vi "bigcryo_Harry-IcT - v2.vi"(10 "Stop":bool, 11 "Measure":bool) -> ()   [LabVIEW 2019]
uses:
  Components/Global 2.vi
  <vilib>/Utility/file.llb/Read From Spreadsheet File (DBL).vi
panel:
  out "SampleTemp":dbl
  in  "Settle Time (s)":dbl=60.0
  in  "Step/Ramp":bool=TRUE
  in  "T Rate (K/min)":dbl=0.1
  out "dV/dI-I":cluster{dbl[], dbl[]}(graph) caption="XY Graph"
  out "I-V":cluster{dbl[], dbl[]}(graph) caption="XY Graph"
  out "Status":string="Measuring..."
  in  "Keithley":refnum<visa-resource-name>="GPIB1::20::INSTR"
  in  "Delay [sec]":dbl=0.002 format="%#_6e"
  in  "Compliance [V] 2":dbl=10.0 format="%#_6f"
  in  "Delta [A]":dbl=1e-05 format="%#_6e"
  in  "Abort Conductance":bool
  in  "Step [A]":dbl=1e-05 format="%#_6e"
  in  "I-Max [A]":dbl=0.002 format="%#_6e"
  in  "Arm Conductance":bool
  in  "Directory Output":string="C:\\User Data\\hlb54\\210111_42B\\JJ1\\IcT_test"
  in  "Minicryo":bool=TRUE
  in  "Field and rate":dbl[][](array[numeric])
  out "?":refnum<visa-resource-name>="GPIB1::20::INSTR"
  out "Iteration?":i32=401
  in  "Start Temp (K)":dbl=2.0 format="%#_7f"
  in  "T Step (K)":dbl=0.01
  out "T Aim":dbl=2.02
  in  "Stop Temp (K)":dbl=2.1
  # "Step"
  # "Ramp"
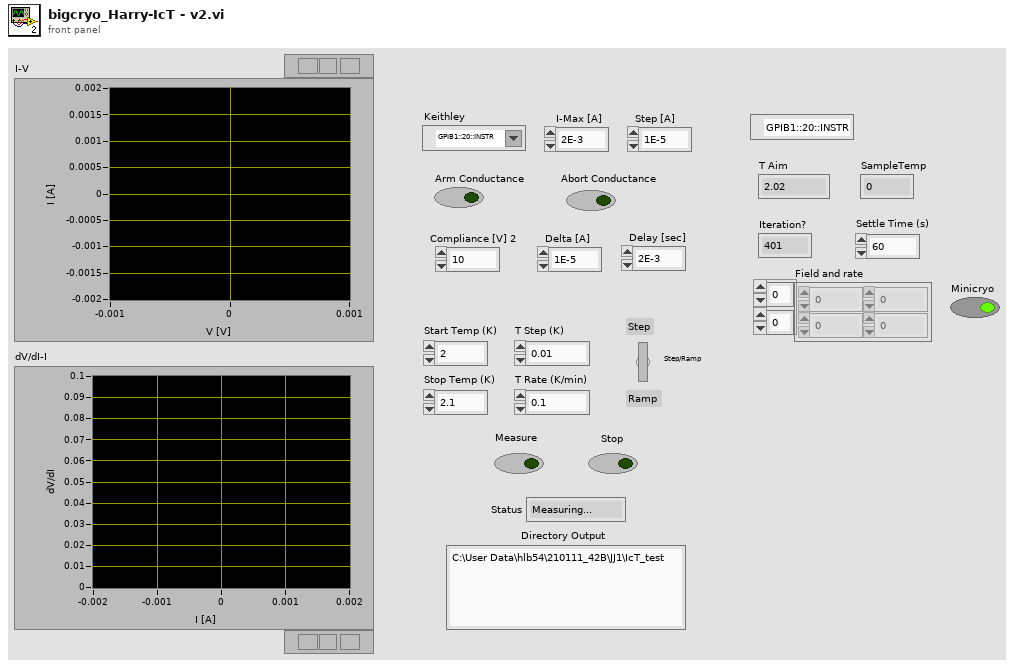
[diagram p1: front panel]
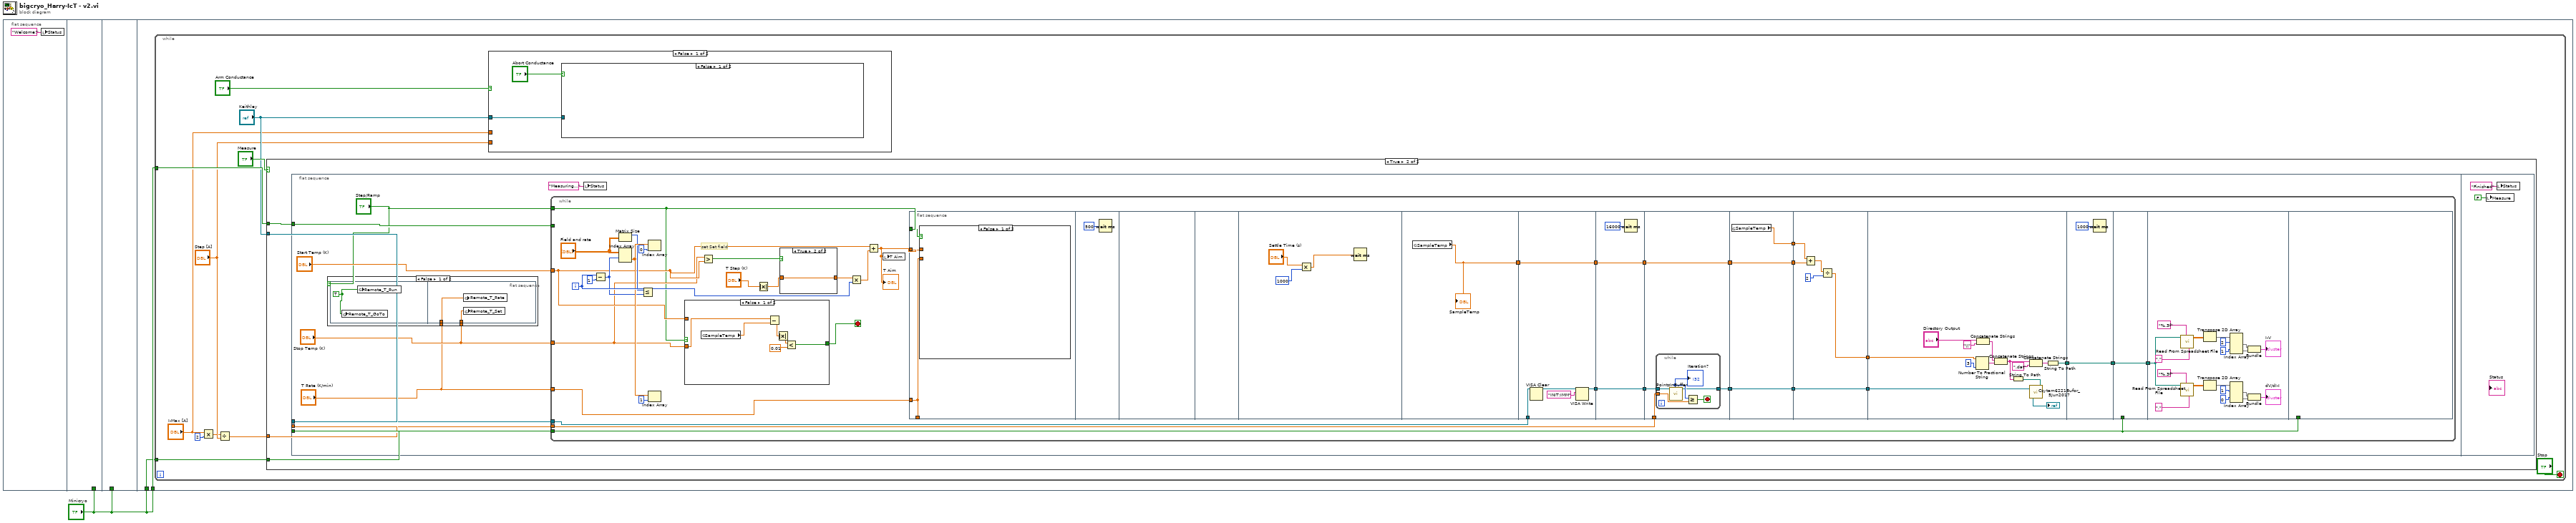
[diagram p0: block diagram]
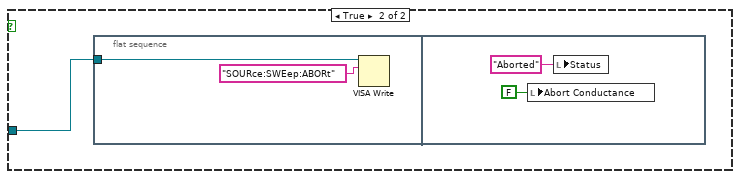
[diagram p2: hidden frame]
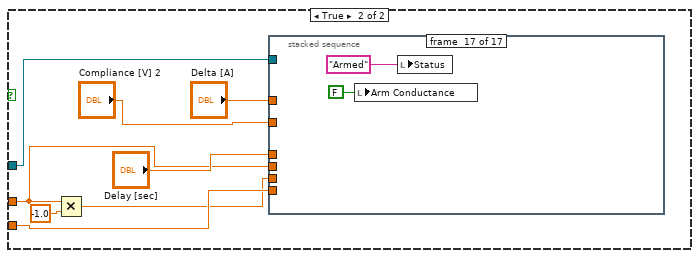
[diagram p3: hidden frame]
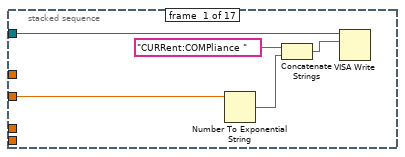
[diagram p4: hidden frame]
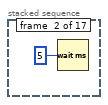
[diagram p5: hidden frame]
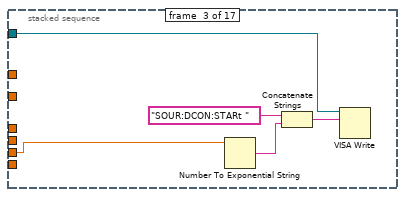
[diagram p6: hidden frame]
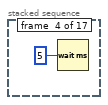
[diagram p7: hidden frame]
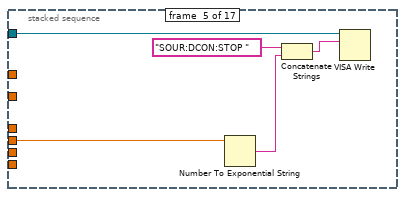
[diagram p8: hidden frame]
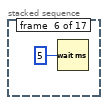
[diagram p9: hidden frame]
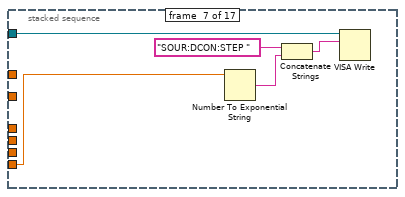
[diagram p10: hidden frame]
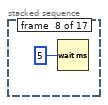
[diagram p11: hidden frame]
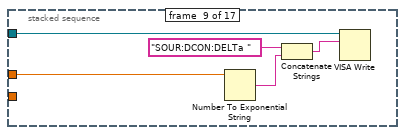
[diagram p12: hidden frame]
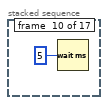
[diagram p13: hidden frame]
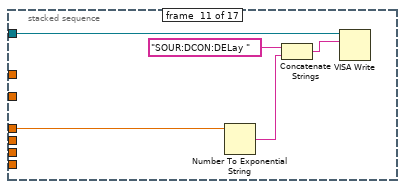
[diagram p14: hidden frame]
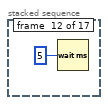
[diagram p15: hidden frame]
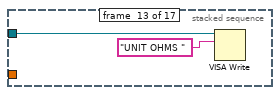
[diagram p16: hidden frame]
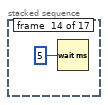
[diagram p17: hidden frame]
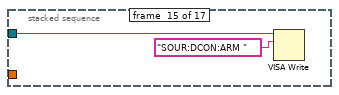
[diagram p18: hidden frame]
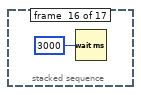
[diagram p19: hidden frame]
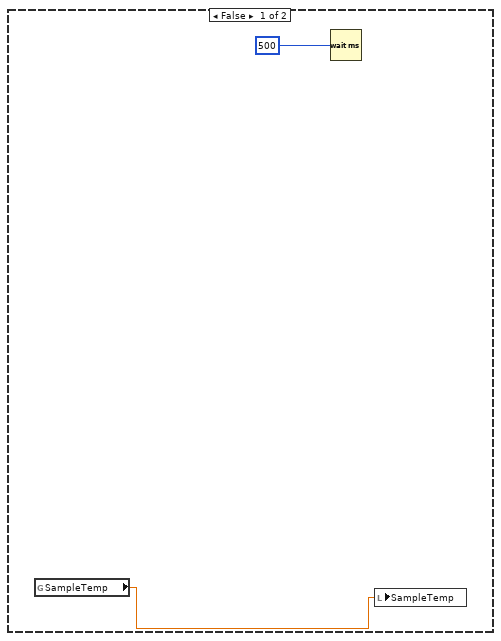
[diagram p20: hidden frame]
diagram:
  n1 = flat-sequence {
    tunnel: "Minicryo" -> [_]
    tunnel: "Minicryo" -> [_]
    tunnel: "Minicryo" -> [w4]
    tunnel: "Minicryo" -> [w3]
    frame #0 {
      n2 = local write "Status"("Welcome!") -> ()
    }
    frame #1 {
    }
    frame #2 {
    }
    frame #3 {
      n3 = while {
        tunnel: w4 -> [w15]
        tunnel: w3 -> [w14]
        stop <- "Stop" stop-if-true
        n4 = Multiply(x="I-Max [A]", y=2) -> (x*y=w5:dbl)
        n5 = Divide(x=w5, y="Step [A]") -> (x/y=w6:dbl)
        n6 = case shown="True" "Measure" {
          tunnel: w15 -> [_ w80]
          tunnel: w14 -> [_ w79]
          tunnel: "Keithley" -> [_ w78]
          tunnel: w6 -> [_ w77]
          frame False {
            n7 = global read "Global 2.vi" "SampleTemp"() -> (w75:dbl)
            n8 = Wait (ms)(milliseconds to wait=u32 500) -> ()  [unwired: 1 out]
            n9 = local write "SampleTemp"(w75) -> ()
          }
          frame True {
            n10 = flat-sequence {
              tunnel: w80 -> [w89]
              tunnel: w79 -> [w88]
              tunnel: w78 -> [w87]
              tunnel: w77 -> [w86]
              frame #0 {
                n11 = case shown="False" "Step/Ramp" {
                  tunnel: "Stop Temp (K)" -> [w91 _]
                  tunnel: "T Rate (K/min)" -> [w90 _]
                  frame False {
                    n12 = flat-sequence {
                      tunnel: w91 -> [w94]
                      tunnel: w90 -> [w93]
                      frame #0 {
                        w92 = TRUE
                        n13 = global write "Global 2.vi" "Remote_T_GoTo"(w92) -> ()
                        n14 = global write "Global 2.vi" "Remote_T_Run"(w92) -> ()
                      }
                      frame #1 {
                        n15 = global write "Global 2.vi" "Remote_T_Rate"(w93) -> ()
                        n16 = global write "Global 2.vi" "Remote_T_Set"(w94) -> ()
                      }
                    }
                  }
                  frame True {
                  }
                }
                n17 = while {
                  tunnel: w89 -> [_]
                  tunnel: w88 -> [w120]
                  tunnel: w87 -> [w119]
                  tunnel: w86 -> [w118]
                  tunnel: "Step/Ramp" -> [w95]
                  tunnel: "Start Temp (K)" -> [w103]
                  tunnel: "Stop Temp (K)" -> [w102]
                  tunnel: "T Rate (K/min)" -> [w101]
                  i -> [w127]
                  stop <- w117 stop-if-true
                  # "set Set field"
                  n18 = Subtract(x=w127, y=1) -> (x-y=w121:i32)
                  n19 = Matrix Size(0:"Field and rate") -> (1:w122:i32)  [unwired: 1 out]
                  n20 = Index Array(array="Field and rate", index (row)=w121) -> (element=w124:dbl[])  [unwired: 1 in]
                  n21 = Less Or Equal?(x=w122, y=w121) -> ()  [unwired: 1 out]
                  n22 = Index Array(array=w124, index=0) -> ()  [unwired: 1 out]
                  n23 = Index Array(array=w124, index=1) -> ()  [unwired: 1 out]
                  n24 = case shown="False" w95 {
                    tunnel: [w134 w142] -> w117
                    tunnel: w103 -> [_ w141]
                    tunnel: w102 -> [w132 w140]
                    frame False {
                      n25 = global read "Global 2.vi" "SampleTemp"() -> (w133:dbl)
                      n26 = Subtract(x=w132, y=w133) -> (x-y=w137:dbl)
                      n27 = Absolute Value(x=w137) -> (abs(x)=w136:dbl)
                      n28 = Less?(x=w136, y=0.01) -> (x < y?=w134:bool)
                    }
                    frame True {
                      n29 = Greater?(x=w140, y=w141) -> (0:w138:bool)
                      n30 = local read "T Aim"() -> (w139:dbl)
                      n31 = case shown="True" w138 {
                        tunnel: [w145 w148] -> w142
                        tunnel: w139 -> [w143 w147]
                        tunnel: w140 -> [w144 w146]
                        frame False {
                          n32 = Less Or Equal?(x=w143, y=w144) -> (x <= y?=w145:bool)
                        }
                        frame True {
                          n33 = Greater Or Equal?(x=w147, y=w146) -> (x >= y?=w148:bool)
                        }
                      }
                    }
                  }
                  n34 = Greater?(x=w102, y=w103) -> (0:w96:bool)
                  n35 = Absolute Value(x="T Step (K)") -> (abs(x)=w98:dbl)
                  n36 = case shown="True" w96 {
                    tunnel: [w151 w152] -> w97
                    tunnel: w98 -> [w149 w152]
                    frame False {
                      n37 = Multiply(x=w149, y=-1) -> (x*y=w151:dbl)
                    }
                    frame True {
                    }
                  }
                  n38 = Multiply(x=w97, y=w127) -> (x*y=w100:dbl)
                  n39 = Add(x=w103, y=w100) -> (x+y=w131:dbl)
                  "T Aim" <- w131
                  n40 = local write "T Aim"(w131) -> ()
                  n41 = flat-sequence {
                    tunnel: w131 -> [w155]
                    tunnel: [w154] -> _
                    tunnel: w101 -> [w154]
                    tunnel: w95 -> [w153]
                    tunnel: [w163] -> w109
                    tunnel: [w166] -> w129
                    tunnel: w119 -> [w165]
                    tunnel: w109 -> [w164]
                    tunnel: [w164] -> w108
                    tunnel: [w171] -> w130
                    tunnel: w129 -> [w171]
                    tunnel: w108 -> [w169]
                    tunnel: [w169] -> w107
                    tunnel: w130 -> [w175]
                    tunnel: [w174] -> w113
                    tunnel: w118 -> [w173]
                    tunnel: w107 -> [w172]
                    tunnel: [w172] -> w106
                    tunnel: w113 -> [w183]
                    tunnel: [w183] -> w112
                    tunnel: [w181] -> w110
                    tunnel: w106 -> [w182]
                    tunnel: [w182] -> w105
                    tunnel: w112 -> [w189]
                    tunnel: [w189] -> w111
                    tunnel: w110 -> [w186]
                    tunnel: w105 -> [w185]
                    tunnel: [w184] -> w104
                    tunnel: w111 -> [w198]
                    tunnel: [w194] -> w114
                    tunnel: w104 -> [w190]
                    tunnel: [w203] -> w115
                    tunnel: w114 -> [w203]
                    tunnel: w120 -> [_]
                    tunnel: [w205] -> w116
                    tunnel: w115 -> [w205]
                    tunnel: w116 -> [w206]
                    tunnel: w120 -> [_]
                    frame #0 {
                      n42 = case shown="False" w153 {
                        tunnel: w155 -> [_ w157]
                        tunnel: w154 -> [_ w158]
                        frame False {
                        }
                        frame True {
                          w156 = TRUE
                          n43 = global write "Global 2.vi" "Remote_T_GoTo"(w156) -> ()
                          n44 = global write "Global 2.vi" "Remote_T_Run"(w156) -> ()
                          n45 = global write "Global 2.vi" "Remote_T_Ramp"(w156) -> ()
                          n46 = global write "Global 2.vi" "Remote_T_Rate"(w158) -> ()
                          n47 = global write "Global 2.vi" "Remote_T_Set"(w157) -> ()
                        }
                      }
                    }
                    frame #1 {
                      n48 = Wait (ms)(milliseconds to wait=u32 500) -> ()  [unwired: 1 out]
                    }
                    frame #2 {
                    }
                    frame #3 {
                    }
                    frame #4 {
                      n49 = Multiply(x="Settle Time (s)", y=1000) -> (x*y=w162:dbl)
                      n50 = Wait (ms)(milliseconds to wait=w162) -> ()  [unwired: 1 out]
                    }
                    frame #5 {
                      n51 = global read "Global 2.vi" "SampleTemp"() -> (w163:dbl)
                      "SampleTemp" <- w163
                    }
                    frame #6 {
                      n52 = VISA Clear(VISA resource name=w165) -> (VISA resource name out=w168:refnum<visa-resource-name>)  [unwired: 1 in, 1 out]
                      n53 = VISA Write(VISA resource name=w168, write buffer="INIT:IMM") -> (VISA resource name out=w166:refnum<visa-resource-name>)  [unwired: 1 in, 2 out]
                    }
                    frame #7 {
                      n54 = Wait (ms)(milliseconds to wait=16000) -> ()  [unwired: 1 out]
                    }
                    frame #8 {
                      n55 = while {
                        tunnel: w175 -> [w178]
                        tunnel: [w177] -> w174
                        tunnel: w173 -> [w176]
                        stop <- w179 stop-if-true
                        n56 = call "PointsInBuffer.vi"("VISA resource name"=w178) -> (3:w177:refnum<visa-resource-name>, "number"=w180:i32)  [unwired: 9 in]
                        "Iteration?" <- w180
                        n57 = Greater Or Equal?(x=w180, y=w176) -> (x >= y?=w179:bool)
                      }
                    }
                    frame #9 {
                      n58 = global read "Global 2.vi" "SampleTemp"() -> (w181:dbl)
                    }
                    frame #10 {
                      n59 = Add(x=w186, y=w185) -> (x+y=w187:dbl)
                      n60 = Divide(x=w187, y=2) -> (x/y=w184:dbl)
                    }
                    frame #11 {
                      n61 = Number To Fractional String(number=w190, precision (6)=i16 3) -> (F-format string=w202:string)  [unwired: 2 in]
                      n62 = Concatenate Strings("Directory Output", "\\") -> (w191:string)
                      n63 = Concatenate Strings(w191, w202) -> (w196:string)
                      n64 = String To Path(string=w196) -> (path=w201:path)
                      n65 = Concatenate Strings(w196, ".dat") -> (w195:string)
                      n66 = call "Czytam6221Bufor_5Jun2017.vi"("file path (dialog if empty)"=w201, 3:w198) -> (2:→"?":refnum<visa-resource-name>)  [unwired: 1 in]
                      n67 = String To Path(string=w195) -> (path=w194:path)
                    }
                    frame #12 {
                      n68 = Wait (ms)(milliseconds to wait=u32 1000) -> ()  [unwired: 1 out]
                    }
                    frame #13 {
                    }
                    frame #14 {
                      n69 = call-poly <vilib>:"Read From Spreadsheet File.vi"("delimiter (\\t)"="," ("delimiter (\\t)"), "format (%.3f)"="%.3f", "file path (dialog if empty)"=w206) -> ("all rows"=w219:dbl[][])  [unwired: 4 in, 4 out]
                      n70 = call-poly <vilib>:"Read From Spreadsheet File.vi"("delimiter (\\t)"="," ("delimiter (\\t)"), "format (%.3f)"="%.3f", "file path (dialog if empty)"=w206) -> ("all rows"=w210:dbl[][])  [unwired: 4 in, 4 out]
                      n71 = Transpose 2D Array(2D array=w219) -> (transposed array=w218:dbl[][])
                      n72 = Transpose 2D Array(2D array=w210) -> (transposed array=w209:dbl[][])
                      n73 = Index Array(array=w218, index (row) #1=2 ("index (row)"), index (row) #2=1 ("index (row)")) -> (element #1=w221:dbl[], element #2=w220:dbl[])  [unwired: 2 in]
                      n74 = Index Array(array=w209, index (row) #1=1 ("index (row)"), index (row) #2=0 ("index (row)")) -> (element #1=w212:dbl[], element #2=w211:dbl[])  [unwired: 2 in]
                      n75 = Bundle(w221, w220) -> (→"I-V":cluster{dbl[], dbl[]})  [unwired: 1 in]
                      n76 = Bundle(w212, w211) -> (→"dV/dI-I":cluster{dbl[], dbl[]})  [unwired: 1 in]
                    }
                    frame #15 {
                    }
                  }
                }
                n77 = local write "Status"("Measuring...") -> ()
              }
              frame #1 {
                n78 = local write "Measure"(FALSE) -> ()
                n79 = local write "Status"("Finished") -> ()
              }
            }
          }
        }
        n80 = case shown="False" "Arm Conductance" {
          tunnel: "Keithley" -> [w16 w26]
          tunnel: "Step [A]" -> [_ w25]
          tunnel: "I-Max [A]" -> [_ w23]
          frame False {
            n81 = case shown="False" "Abort Conductance" {
              tunnel: w16 -> [_ w18]
              frame False {
              }
              frame True {
                n82 = flat-sequence {
                  tunnel: w18 -> [w19]
                  frame #0 {
                    n83 = VISA Write(VISA resource name=w19, write buffer="SOURce:SWEep:ABORt") -> ()  [unwired: 1 in, 3 out]
                  }
                  frame #1 {
                    n84 = local write "Abort Conductance"(FALSE) -> ()
                    n85 = local write "Status"("Aborted") -> ()
                  }
                }
              }
            }
          }
          frame True {
            n86 = Multiply(x=w23, y=-1.0) -> (x*y=w24:dbl)
            n87 = stacked-sequence {
              tunnel: w24 -> [_ _ w39 _ _ _ _ _ _ _ _ _ _ _ _ _ _]
              tunnel: "Delay [sec]" -> [_ _ _ _ _ _ _ _ _ _ w62 _ _ _ _ _ _]
              tunnel: "Compliance [V] 2" -> [w32 _ _ _ _ _ _ _ _ _ _ _ _ _ _ _ _]
              tunnel: "Delta [A]" -> [_ _ _ _ _ _ _ _ w56 _ _ _ _ _ _ _ _]
              tunnel: w26 -> [w31 _ w37 _ w44 _ w50 _ w55 _ w61 _ w67 _ w70 _ _]
              tunnel: w25 -> [_ _ _ _ _ _ w49 _ _ _ _ _ _ _ _ _ _]
              tunnel: w23 -> [_ _ _ _ w43 _ _ _ _ _ _ _ _ _ _ _ _]
              frame #0 {
                n88 = Number To Exponential String(number=w32) -> (E-format string=w34:string)  [unwired: 3 in]
                n89 = Concatenate Strings("CURRent:COMPliance ", w34) -> (w33:string)
                n90 = VISA Write(VISA resource name=w31, write buffer=w33) -> ()  [unwired: 1 in, 3 out]
              }
              frame #1 {
                n91 = Wait (ms)(milliseconds to wait=5) -> ()  [unwired: 1 out]
              }
              frame #2 {
                n92 = Number To Exponential String(number=w39) -> (E-format string=w40:string)  [unwired: 3 in]
                n93 = Concatenate Strings("SOUR:DCON:STARt ", w40) -> (w38:string)
                n94 = VISA Write(VISA resource name=w37, write buffer=w38) -> ()  [unwired: 1 in, 3 out]
              }
              frame #3 {
                n95 = Wait (ms)(milliseconds to wait=5) -> ()  [unwired: 1 out]
              }
              frame #4 {
                n96 = Number To Exponential String(number=w43) -> (E-format string=w46:string)  [unwired: 3 in]
                n97 = Concatenate Strings("SOUR:DCON:STOP ", w46) -> (w45:string)
                n98 = VISA Write(VISA resource name=w44, write buffer=w45) -> ()  [unwired: 1 in, 3 out]
              }
              frame #5 {
                n99 = Wait (ms)(milliseconds to wait=5) -> ()  [unwired: 1 out]
              }
              frame #6 {
                n100 = Number To Exponential String(number=w49) -> (E-format string=w52:string)  [unwired: 3 in]
                n101 = Concatenate Strings("SOUR:DCON:STEP ", w52) -> (w51:string)
                n102 = VISA Write(VISA resource name=w50, write buffer=w51) -> ()  [unwired: 1 in, 3 out]
              }
              frame #7 {
                n103 = Wait (ms)(milliseconds to wait=5) -> ()  [unwired: 1 out]
              }
              frame #8 {
                n104 = Number To Exponential String(number=w56) -> (E-format string=w58:string)  [unwired: 3 in]
                n105 = Concatenate Strings("SOUR:DCON:DELTa ", w58) -> (w57:string)
                n106 = VISA Write(VISA resource name=w55, write buffer=w57) -> ()  [unwired: 1 in, 3 out]
              }
              frame #9 {
                n107 = Wait (ms)(milliseconds to wait=5) -> ()  [unwired: 1 out]
              }
              frame #10 {
                n108 = Number To Exponential String(number=w62) -> (E-format string=w64:string)  [unwired: 3 in]
                n109 = Concatenate Strings("SOUR:DCON:DELay ", w64) -> (w63:string)
                n110 = VISA Write(VISA resource name=w61, write buffer=w63) -> ()  [unwired: 1 in, 3 out]
              }
              frame #11 {
                n111 = Wait (ms)(milliseconds to wait=5) -> ()  [unwired: 1 out]
              }
              frame #12 {
                n112 = VISA Write(VISA resource name=w67, write buffer="UNIT OHMS ") -> ()  [unwired: 1 in, 3 out]
              }
              frame #13 {
                n113 = Wait (ms)(milliseconds to wait=5) -> ()  [unwired: 1 out]
              }
              frame #14 {
                n114 = VISA Write(VISA resource name=w70, write buffer="SOUR:DCON:ARM ") -> ()  [unwired: 1 in, 3 out]
              }
              frame #15 {
                n115 = Wait (ms)(milliseconds to wait=3000) -> ()  [unwired: 1 out]
              }
              frame #16 {
                n116 = local write "Arm Conductance"(FALSE) -> ()
                n117 = local write "Status"("Armed") -> ()
              }
            }
          }
        }
      }
    }
  }
